vi "PH meter.vi"(1 "통신포트":refnum<visa-resource-name>="COM8") -> ()   [LabVIEW 2018]
uses:
  <vilib>/Instr/_visa.llb/VISA Configure Serial Port (Instr).vi
panel:
  out "PH":dbl format="%#.2g"
  out "웨이브폼 차트":dbl(graph)
  in  "정지":bool
  # "PH meter (E201-BNC)"
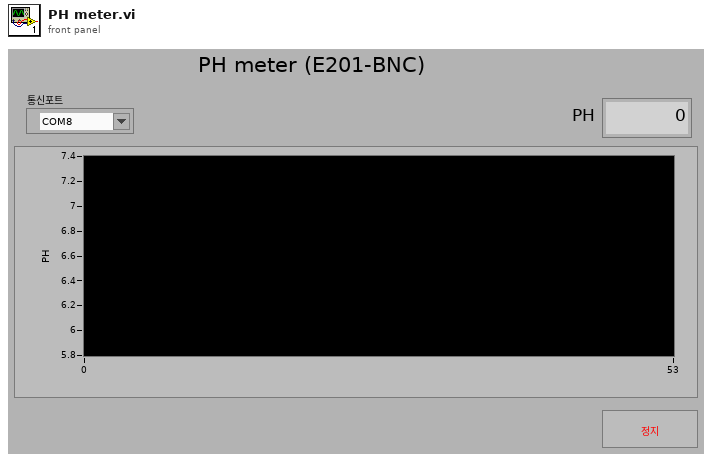
[diagram p1: front panel]
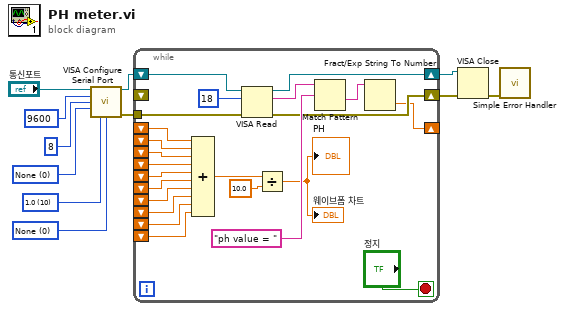
[diagram p0: block diagram]
diagram:
  w7 = u16 0 items=["None"=0, "XON/XOFF"=1, "RTS/CTS"=2, "DTR/DSR"=4] ("flow control")
  w8 = u16 10 items=["1.0"=10, "1.5"=15, "2.0"=20] ("stop bits")
  w9 = u16 0 items=["None", "Odd", "Even", "Mark", "Space"] ("parity")
  n1 = call-poly "VISA Configure Serial Port"("VISA resource name"="통신포트", "baud rate (9600)"=u32 9600 ("baud rate"), "data bits (8)"=u16 8 ("data bits"), "parity (0:none)"=w9, "stop bits (10: 1 bit)"=w8, "flow control (0:none)"=w7) -> ("VISA resource name out"=w5:refnum<visa-resource-name>, "error out"=w4:errorcluster)  [unwired: 8 in]
  n2 = while {
    tunnel: w4 -> [w32]
    shift-right: [w27] -> w2
    shift-left: w5 -> [w33]
    shift-right: [w26] -> w1
    shift-left: _ -> [_]
    shift-right: [w25] -> _
    shift-left: _ -> [w24]
    shift-left: _ -> [w23]
    shift-left: _ -> [w22]
    shift-left: _ -> [w21]
    shift-left: _ -> [w20]
    shift-left: _ -> [w16]
    shift-left: _ -> [w15]
    shift-left: _ -> [w14]
    shift-left: _ -> [w13]
    shift-left: _ -> [w12]
    stop <- "정지" stop-if-true
    n3 = Compound Arithmetic op=ADD(w24, w23, w22, w21, w20, w16, w15, w14, w13, w12) -> (w19:dbl)
    n4 = VISA Read(VISA resource name=w33, byte count=u32 18 ("바이트 카운트"), error in (no error)=w32) -> (VISA resource name out=w27:refnum<visa-resource-name>, read buffer=w30:string, error out=w26:errorcluster)  [unwired: 1 out]
    n5 = Divide(x=w19, y=10.0) -> (x/y=→"웨이브폼 차트" →"PH":dbl)
    n6 = Match Pattern(string=w30, regular expression="ph value = " ("검색 문자열")) -> (after substring=w28:string)  [unwired: 1 in, 3 out]
    n7 = Fract/Exp String To Number(string=w28) -> (number=w25:dbl)  [unwired: 3 in, 1 out]
  }
  n8 = VISA Close(VISA resource name=w2, error in (no error)=w1) -> (error out=w3:errorcluster)
  n9 = call <vilib>:"Simple Error Handler.vi"("error in (no error)"=w3) -> ()  [unwired: 4 in, 5 out]
